vi "MICSD Receive MICS Data.vi"(8 "error in (no error)":errorcluster, 9 "Timeout(mS)":dbl=3000.0, 10 "BlockSize":u8=15, 11 "VISA Resource Name":refnum<visa-resource-name>) -> (0 "error out":errorcluster, 1 "Bytes Remaining?":bool, 2 "Receive Data":u8[](array[numeric]) format="%02x", 3 "dup VISA Resource Name":refnum<visa-resource-name>)   [LabVIEW 2020]
uses:
  <vilib>/Instr/_visa.llb/VISA Configure Serial Port (Instr).vi
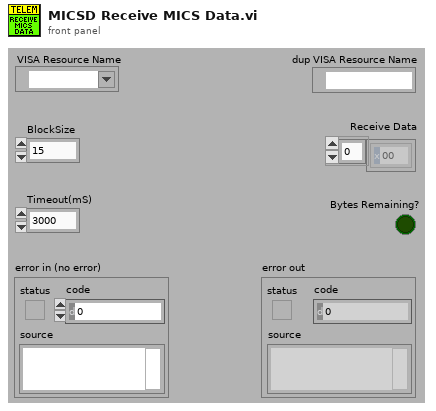
[diagram p1: front panel]
types:
  T1 = cluster{"Command Token":u8, "Length":u16, "Pack Data":u8[]}
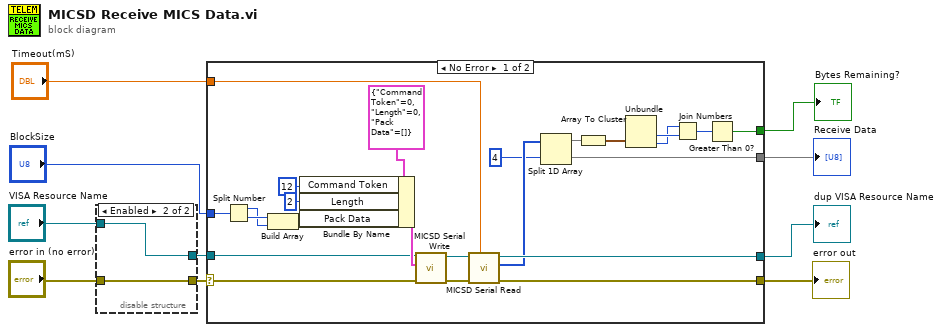
[diagram p0: block diagram]
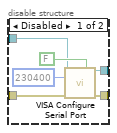
[diagram p2: hidden frame]
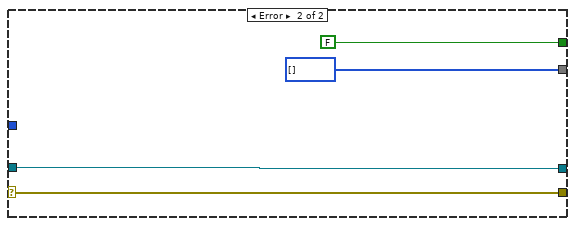
[diagram p3: hidden frame]
diagram:
  n1 = disable-structure shown="Enabled" {
    disable-tunnel: [w14 w17] -> w10
    disable-tunnel: [w13 w18] -> w9
    disable-tunnel: "VISA Resource Name" -> [w12 w18]
    disable-tunnel: "error in (no error)" -> [w11 w17]
    frame Disabled {
      n2 = call-poly "VISA Configure Serial Port"("VISA resource name"=w12, "Enable Termination\nChar (T)"=FALSE ("Enable Termination\nChar (T)"), "baud rate (9600)"=u32 230400, "error in (no error)"=w11) -> ("VISA resource name out"=w13:refnum<visa-resource-name>, "error out"=w14:errorcluster)  [unwired: 10 in]
    }
    frame Enabled {
    }
  }
  n3 = case shown="No Error" w10 {
    selector: w10 -> [w20 w46]
    tunnel: [w37 w46] -> w5
    tunnel: w9 -> [w21 w45]
    tunnel: [w36 w45] -> w6
    tunnel: [w28 u8[] []] -> w4
    tunnel: "BlockSize" -> [w30 _]
    tunnel: [w22 FALSE] -> w2
    tunnel: "Timeout(mS)" -> [w19 _]
    frame No Error {
      n4 = Split Number(x=w30) -> (hi(x)=w31:u8, lo(x)=w32:u8)
      n5 = Build Array(w32, w31) -> (w33:u8[])
      n6 = Bundle By Name(cluster=T1 {"Command Token"=0, "Length"=0, "Pack Data"=[]} ("Write Data"), "Command Token"=u8 12, "Length"=u16 2, "Pack Data"=w33) -> (w42:T1)
      n7 = call "MICSD Serial Write.vi"("error in (no error)"=w20, "Write Data"=w42, "VISA Resource Name"=w21) -> ("error out"=w35:errorcluster, "DUP Visa Resource Name"=w40:refnum<visa-resource-name>)  [unwired: 7 in]
      n8 = call "MICSD Serial Read.vi"("Timeout(mS)"=w19, "error in (no error)"=w35, "VISA Resource Name"=w40) -> ("error out"=w37:errorcluster, "Read Data"=w34:u8[], "DUP Visa Resource Name"=w36:refnum<visa-resource-name>)  [unwired: 6 in]
      n9 = Split 1D Array(array=w34, index=4) -> (first subarray=w27:u8[], second subarray=w28:u8[])
      n10 = Array To Cluster(array=w27) -> (cluster=w26:cluster{"[0]":u8, "[1]":u8, "[2]":u8, "[3]":u8})
      n11 = Unbundle(w26) -> ("[2]"=w25:u8, "[3]"=w24:u8)  [unwired: 2 out]
      n12 = Join Numbers(hi=w24, lo=w25) -> ((hi.lo)=w23:u16)
      n13 = Greater Than 0?(x=w23) -> (x > 0?=w22:bool)
    }
    frame Error {
    }
  }
  "dup VISA Resource Name" <- w6
  "error out" <- w5
  "Receive Data" <- w4
  "Bytes Remaining?" <- w2
